vi "Panel.vi"(11 "BoardArrayPanel in":refnum<class "BoardArrayPanel.lvclass">) -> ()   [LabVIEW 2020, in "PicoG-App.lvlib" / "BoardArrayPanel.lvclass"]
uses:
  BoardArrayPanel.lvclass
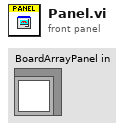
[diagram p1: front panel]
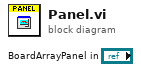
[diagram p0: block diagram]
diagram:
